vi "运维调试_其他.vi"() -> ()   [LabVIEW 2016, in "其他.lvlib"]
uses:
  <vilib>/Utility/miscctls.llb/LVPointTypeDef.ctl
  PLC/PLC.lvlib
  <vilib>/ptbypt/NI_PtbyPt.lvlib
panel:
  out "工作电流":dbl format="%#.2f A"
  out "工作电压":dbl format="%#.2f V"
  out "回风温度":dbl format="%#.2f ℃"
  out "空调通讯状态":u16(ring) items=["通讯异常", "通讯正常"]
  out "送风温度":dbl format="%#.2f ℃"
  out "集成报警信息":string
  out "R115":i16 caption="灯带关闭时间"
  out "R114":i16 caption="灯带开启时间"
  in  "视频监控":bool
  in  "照明":bool
  in  "前门灯带":bool
  in  "侧边灯带":bool
  # "空调运行状态"
  # "H"
  # "H"
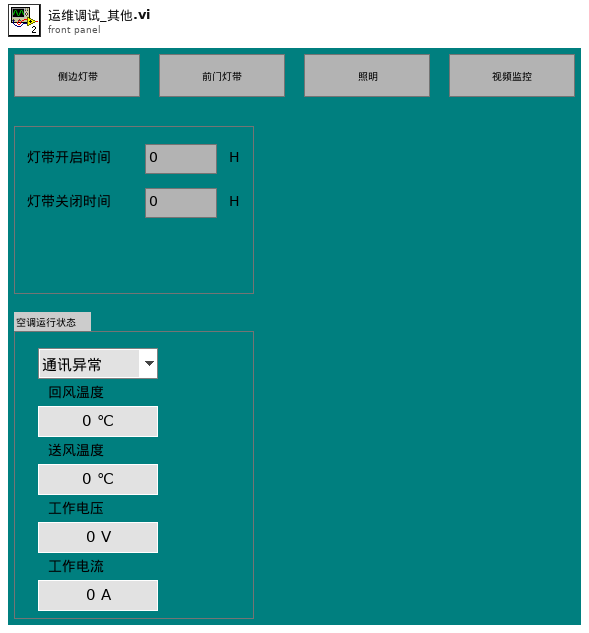
[diagram p1: front panel]
types:
  T1 = cluster{"通讯状态":u16, "回风温度":sgl, "送风温度":sgl, "电压":sgl, "电流":sgl}
  T2 = typedef "LVDateTimeRec.ctl" = cluster{"秒数的小数部分":dbl, "秒":i32, "分":i32, "时":i32, "日":i32, "月":i32, "年":i32, "天数（周）":i32, "天数（年）":i32, "DST":i32}
  T3 = cluster{"时间标识":timestamp, "监测值":sgl, "单位":string}
  T4 = cluster{"R100":i16, "R101":i16, "R102":i16, "R103":i16, "R104":i16, "R105":i16, "R106":i16, "R107":i16, "R108":i16, "R109":i16, "R110":i16, "R111":i16, "R112":i16, "R113":i16, "R114":i16, "R115":i16, "R116":i16, "R117":i16, "R118":i16, "R119":i16}
  T5 = typedef "LVPointTypeDef.ctl" = cluster{"Horizontal":i16, "Vertical":i16}
  T6 = cluster{"命令":string, "data":cluster{"starting address":u16, "coil values":bool[]}}
  T7 = cluster{"命令":string, "数据":cluster{"starting address":u16, "holding register values":u16[]}}
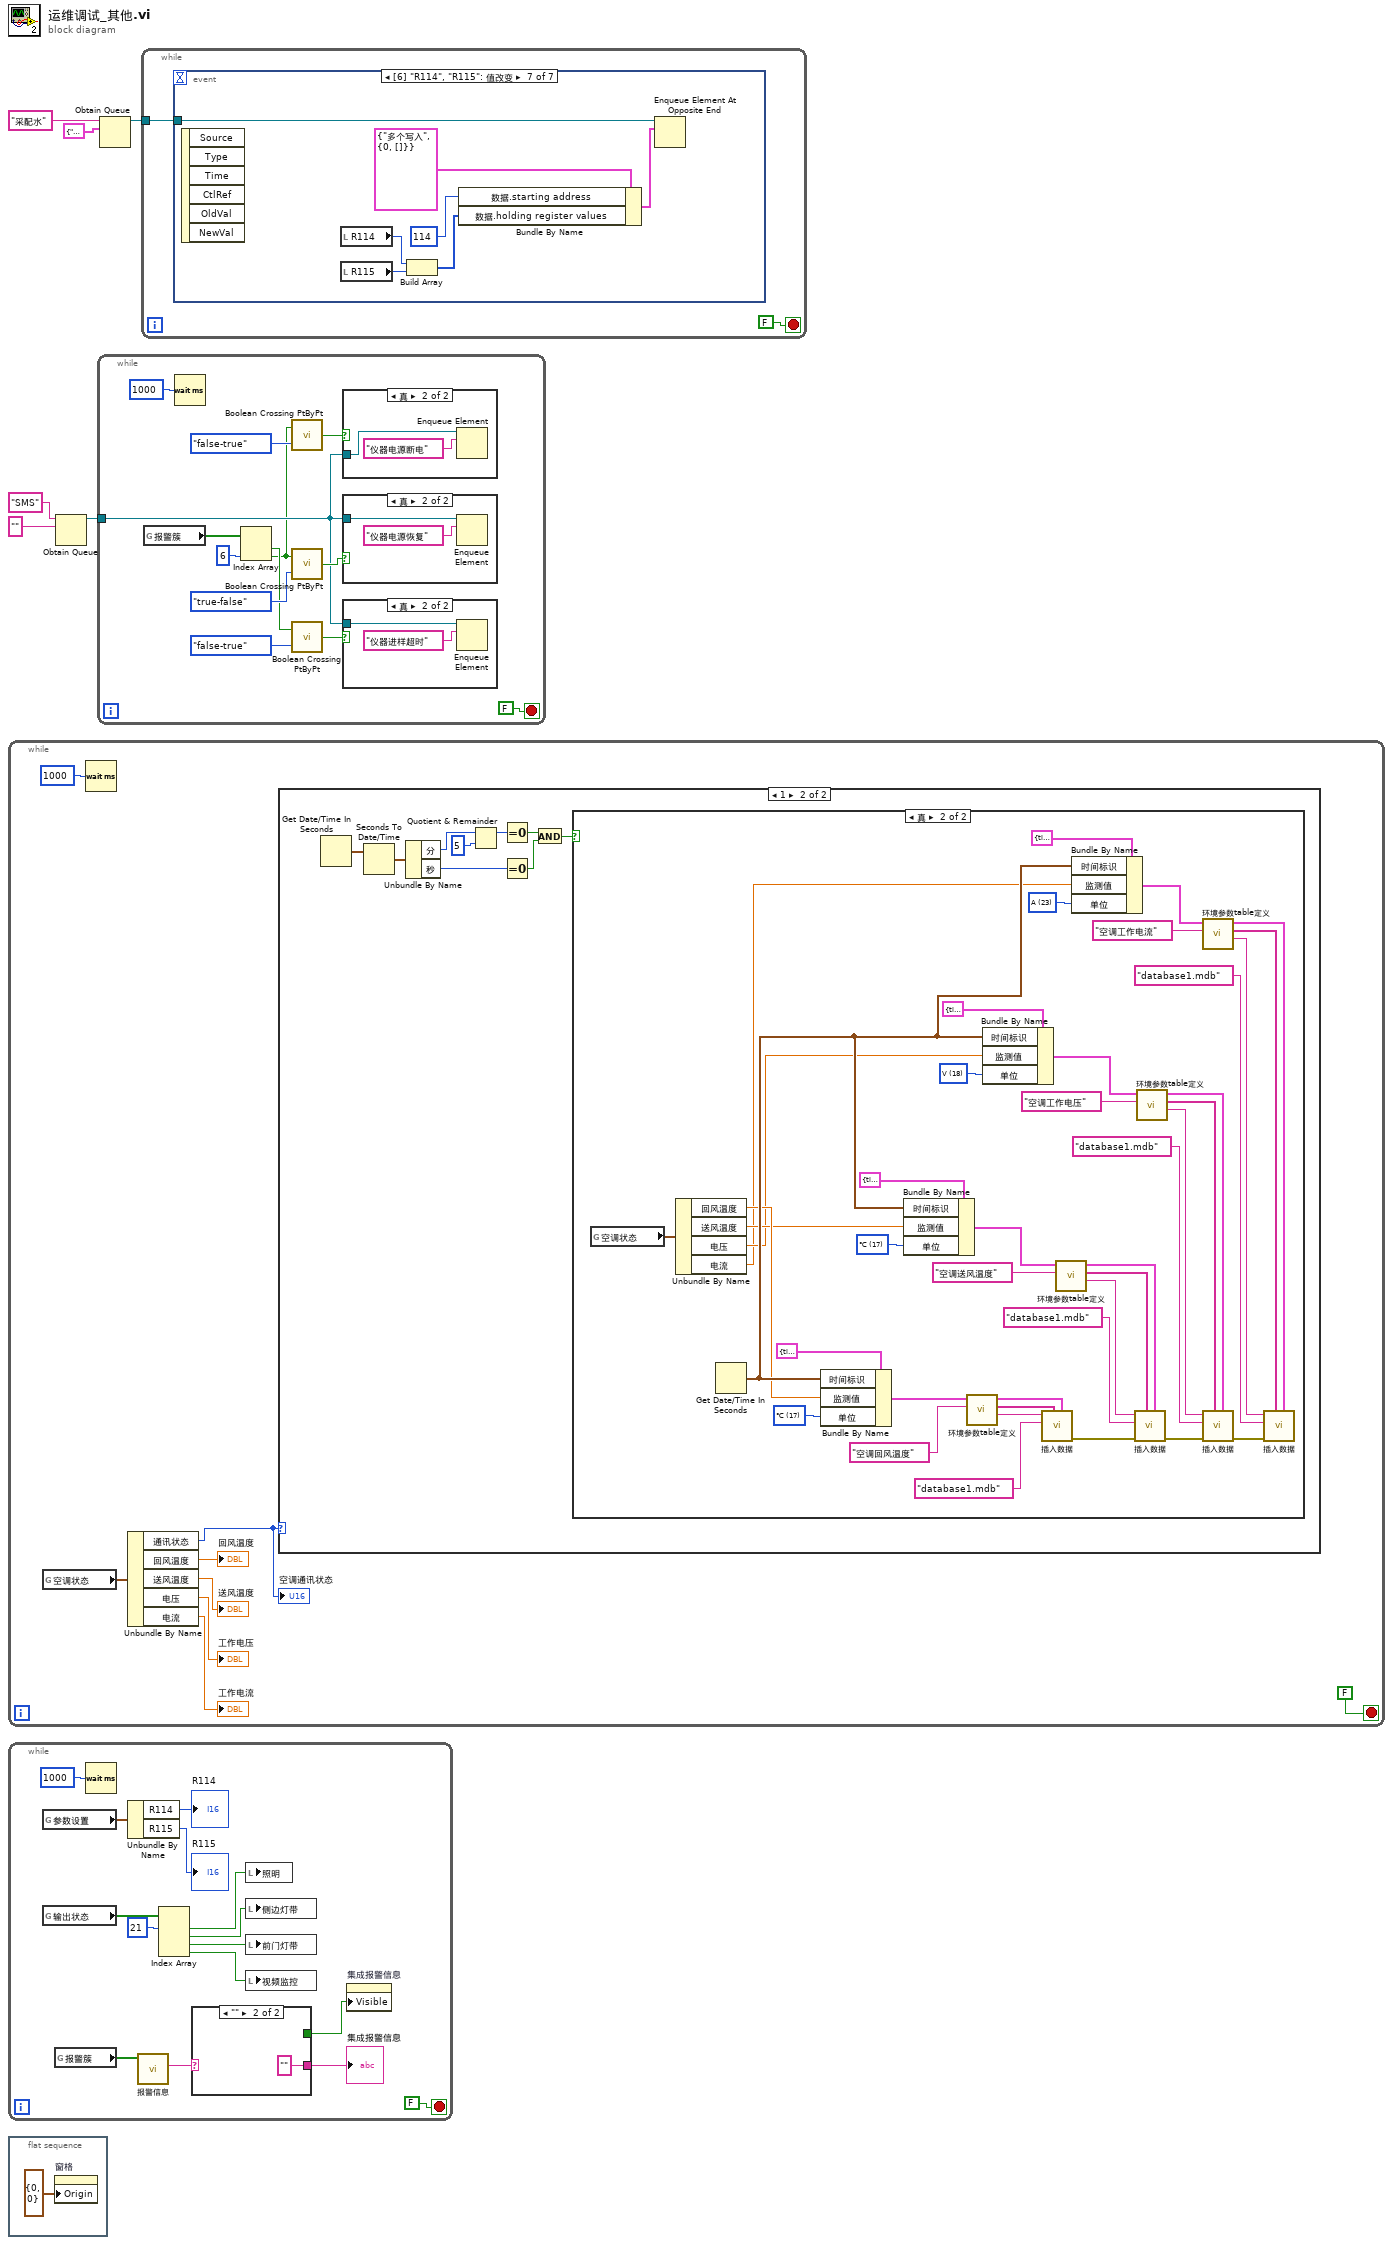
[diagram p0: block diagram]
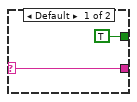
[diagram p7: hidden frame]
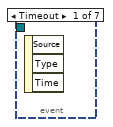
[diagram p8: hidden frame]
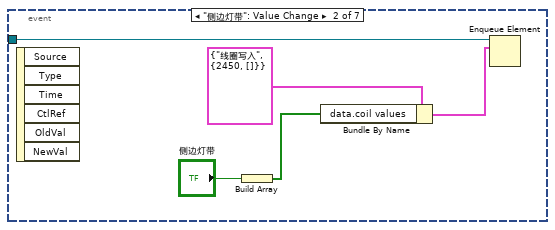
[diagram p9: hidden frame]
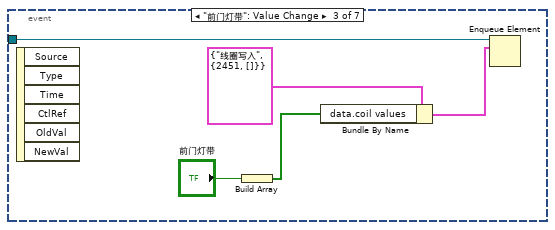
[diagram p10: hidden frame]
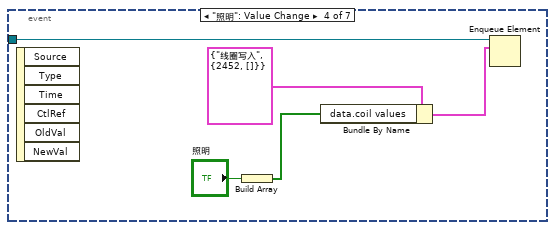
[diagram p11: hidden frame]
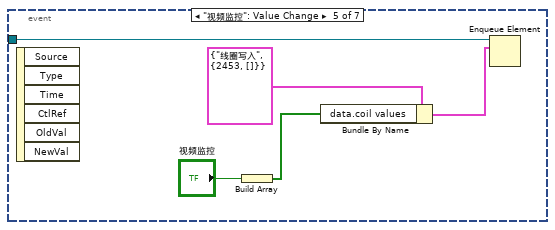
[diagram p12: hidden frame]
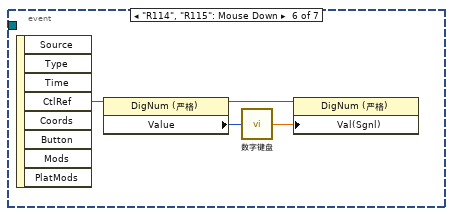
[diagram p13: hidden frame]
diagram:
  n1 = while {
    stop <- FALSE stop-if-true
    n2 = global read "采配水全局变量.vi" "空调状态"() -> (w14:T1)
    n3 = Wait (ms)(milliseconds to wait=u32 1000 ("等待时间（毫秒）")) -> ()  [unwired: 1 out]
    n4 = Unbundle By Name(w14) -> ("通讯状态"=w8:u16, "回风温度"=→"回风温度":sgl, "送风温度"=→"送风温度":sgl, "电压"=→"工作电压":sgl, "电流"=→"工作电流":sgl)
    "空调通讯状态" <- w8
    n5 = case shown="1" w8 {
      frame 0, Default {
      }
      frame 1 {
        n6 = Get Date/Time In Seconds() -> (seconds since 1Jan1904=w23:timestamp)
        n7 = Seconds To Date/Time(time stamp (now)=w23) -> (date time rec=w22:T2)  [unwired: 1 in]
        n8 = Unbundle By Name(w22) -> ("分"=w21:i32, "秒"=w19:i32)
        n9 = Quotient & Remainder(x=w21, y=5) -> (x-y*floor(x/y)=w18:i32)  [unwired: 1 out]
        n10 = Equal To 0?(x=w18) -> (x = 0?=w17:bool)
        n11 = Equal To 0?(x=w19) -> (x = 0?=w16:bool)
        n12 = And(x=w17, y=w16) -> (x .and. y?=w15:bool)
        n13 = case shown="真" w15 {
          frame False {
          }
          frame True {
            w29 = u16 23 items=["ug/L", "mg/L", "ppm", "mg/m3", "cm", "ppb", "ug/m3", "%", "nmol/mol", "umol/mol", "MPN/L", "MPN/100ml", "ng/m3", "NTU", "无量纲", "ms/cm", "us/cm", "℃", "V", "m3/s", "m3", "m", "m/s", "A"] ("单位")
            w45 = u16 18 items=["ug/L", "mg/L", "ppm", "mg/m3", "cm", "ppb", "ug/m3", "%", "nmol/mol", "umol/mol", "MPN/L", "MPN/100ml", "ng/m3", "NTU", "无量纲", "ms/cm", "us/cm", "℃", "V"] ("单位")
            w53 = u16 17 items=["ug/L", "mg/L", "ppm", "mg/m3", "cm", "ppb", "ug/m3", "%", "nmol/mol", "umol/mol", "MPN/L", "MPN/100ml", "ng/m3", "NTU", "无量纲", "ms/cm", "us/cm", "℃", "V"] ("单位")
            w55 = u16 17 items=["ug/L", "mg/L", "ppm", "mg/m3", "cm", "ppb", "ug/m3", "%", "nmol/mol", "umol/mol", "MPN/L", "MPN/100ml", "ng/m3", "NTU", "无量纲", "ms/cm", "us/cm", "℃", "V"] ("单位")
            n14 = global read "采配水全局变量.vi" "空调状态"() -> (w28:T1)
            n15 = Unbundle By Name(w28) -> ("回风温度"=w27:sgl, "送风温度"=w26:sgl, "电压"=w25:sgl, "电流"=w24:sgl)
            n16 = Get Date/Time In Seconds() -> (seconds since 1Jan1904=w30:timestamp)
            n17 = Bundle By Name(cluster=cluster{"时间标识":timestamp, "监测值":sgl, "单位":u16} {"时间标识"=timestamp(0 s since 1904-01-01), "监测值"=0.0, "单位"=0} ("data"), "时间标识"=w30, "监测值"=w27, "单位"=w55) -> (w56:cluster{"时间标识":timestamp, "监测值":sgl, "单位":u16})
            n18 = Bundle By Name(cluster=cluster{"时间标识":timestamp, "监测值":sgl, "单位":u16} {"时间标识"=timestamp(0 s since 1904-01-01), "监测值"=0.0, "单位"=0} ("data"), "时间标识"=w30, "监测值"=w26, "单位"=w53) -> (w52:cluster{"时间标识":timestamp, "监测值":sgl, "单位":u16})
            n19 = call "环境参数table定义.vi"("table 输入"="空调回风温度", "data"=w56) -> ("table 输出"=w64:string, "columns"=w63:string[], "data输出"=w62:T3)  [unwired: 7 in]
            n20 = Bundle By Name(cluster=cluster{"时间标识":timestamp, "监测值":sgl, "单位":u16} {"时间标识"=timestamp(0 s since 1904-01-01), "监测值"=0.0, "单位"=0} ("data"), "时间标识"=w30, "监测值"=w25, "单位"=w45) -> (w44:cluster{"时间标识":timestamp, "监测值":sgl, "单位":u16})
            n21 = call "插入数据.vi"("data"=w62, "columns"=w63, "database"="database1.mdb" ("table 输入"), "table"=w64) -> ("error out"=w58:errorcluster)  [unwired: 7 in]
            n22 = call "环境参数table定义.vi"("table 输入"="空调送风温度", "data"=w52) -> ("table 输出"=w59:string, "columns"=w60:string[], "data输出"=w61:T3)  [unwired: 7 in]
            n23 = Bundle By Name(cluster=cluster{"时间标识":timestamp, "监测值":sgl, "单位":u16} {"时间标识"=timestamp(0 s since 1904-01-01), "监测值"=0.0, "单位"=0} ("data"), "时间标识"=w30, "监测值"=w24, "单位"=w29) -> (w35:cluster{"时间标识":timestamp, "监测值":sgl, "单位":u16})
            n24 = call "插入数据.vi"("data"=w61, "columns"=w60, "error in (no error)"=w58, "database"="database1.mdb" ("table 输入"), "table"=w59) -> ("error out"=w32:errorcluster)  [unwired: 6 in]
            n25 = call "环境参数table定义.vi"("table 输入"="空调工作电压", "data"=w44) -> ("table 输出"=w40:string, "columns"=w41:string[], "data输出"=w42:T3)  [unwired: 7 in]
            n26 = call "环境参数table定义.vi"("table 输入"="空调工作电流", "data"=w35) -> ("table 输出"=w39:string, "columns"=w38:string[], "data输出"=w37:T3)  [unwired: 7 in]
            n27 = call "插入数据.vi"("data"=w42, "columns"=w41, "error in (no error)"=w32, "database"="database1.mdb" ("table 输入"), "table"=w40) -> ("error out"=w31:errorcluster)  [unwired: 6 in]
            n28 = call "插入数据.vi"("data"=w37, "columns"=w38, "error in (no error)"=w31, "database"="database1.mdb" ("table 输入"), "table"=w39) -> ()  [unwired: 6 in, 1 out]
          }
        }
      }
    }
  }
  n29 = while {
    stop <- FALSE stop-if-true
    n30 = global read "采配水全局变量.vi" "参数设置"() -> (w77:T4)
    n31 = global read "采配水全局变量.vi" "输出状态"() -> (w70:bool[])
    n32 = global read "采配水全局变量.vi" "报警簇"() -> (w71:bool[])
    n33 = Wait (ms)(milliseconds to wait=u32 1000 ("等待时间（毫秒）")) -> ()  [unwired: 1 out]
    n34 = Unbundle By Name(w77) -> ("R114"=→"R114":i16, "R115"=→"R115":i16)
    n35 = call "报警信息.vi"("报警簇"=w71) -> ("系统报警信息"=w74:string)  [unwired: 9 in, 1 out]
    n36 = Index Array(array=w70, index #1=21 ("索引")) -> (element #1=w68:bool, element #2=w67:bool, element #3=w69:bool, element #4=w66:bool)  [unwired: 3 in]
    n37 = case shown="\"\"" w74 {
      selector: w74 -> [w81 _]
      tunnel: [w81 "" ("字符串")] -> w72
      tunnel: [TRUE ("可见") _] -> w73
      frame Default {
      }
      frame "" {
      }
    }
    "集成报警信息" <- w72
    n38 = local write "照明"(w68) -> ()
    n39 = local write "侧边灯带"(w67) -> ()
    n40 = local write "前门灯带"(w69) -> ()
    n41 = local write "视频监控"(w66) -> ()
    n42 = property on="集成报警信息" class="Str"("Visible"=w73) -> ()  [unwired: 2 in, 2 out]
  }
  n43 = flat-sequence {
    frame #0 {
      n44 = property on="窗格" class="Pane"("Origin"=T5 {"Horizontal"=0, "Vertical"=0} ("原点")) -> ()  [unwired: 2 in, 2 out]
    }
  }
  n45 = Obtain Queue(name (unnamed)="SMS" ("名称（未命名）"), element data type="" ("名称（未命名）")) -> (queue out=w1:refnum<queue>)  [unwired: 3 in, 2 out]
  n46 = while {
    tunnel: w1 -> [w90]
    stop <- FALSE stop-if-true
    n47 = global read "采配水全局变量.vi" "报警簇"() -> (w87:bool[])
    n48 = Wait (ms)(milliseconds to wait=u32 1000 ("等待时间（毫秒）")) -> ()  [unwired: 1 out]
    n49 = Index Array(array=w87, index #2=6 ("索引")) -> (element #1=w86:bool, element #2=w84:bool)  [unwired: 1 in]
    n50 = call <vilib>:"Boolean Crossing PtByPt.vi"("direction"=enum16{"either", "false-true", "true-false"}."false-true", "input"=w84) -> ("crossing"=w93:bool)  [unwired: 1 in]
    n51 = call <vilib>:"Boolean Crossing PtByPt.vi"("direction"=enum16{"either", "false-true", "true-false"}."true-false", "input"=w84) -> ("crossing"=w91:bool)  [unwired: 1 in]
    n52 = call <vilib>:"Boolean Crossing PtByPt.vi"("direction"=enum16{"either", "false-true", "true-false"}."false-true", "input"=w86) -> ("crossing"=w88:bool)  [unwired: 1 in]
    n53 = case shown="真" w93 {
      tunnel: w90 -> [_ w102]
      frame False {
      }
      frame True {
        n54 = Enqueue Element(queue=w102, element="仪器电源断电" ("元素")) -> ()  [unwired: 2 in, 3 out]
      }
    }
    n55 = case shown="真" w91 {
      tunnel: w90 -> [_ w100]
      frame False {
      }
      frame True {
        n56 = Enqueue Element(queue=w100, element="仪器电源恢复" ("元素")) -> ()  [unwired: 2 in, 3 out]
      }
    }
    n57 = case shown="真" w88 {
      tunnel: w90 -> [_ w98]
      frame False {
      }
      frame True {
        n58 = Enqueue Element(queue=w98, element="仪器进样超时" ("元素")) -> ()  [unwired: 2 in, 3 out]
      }
    }
  }
  n59 = Obtain Queue(name (unnamed)="采配水" ("名称（未命名）"), element data type=cluster{"命令":string, "数据":variant} {"命令"="", "数据"=variant}) -> (queue out=w4:refnum<queue>)  [unwired: 3 in, 2 out]
  n60 = while {
    tunnel: w4 -> [w103]
    stop <- FALSE stop-if-true
    n61 = event shown="[6] \"R114\", \"R115\": 值改变" {
      selector: _ -> [_ _ _ _ _ _ _]
      dyn-events: _ -> [_ _ _ _ _ _ _]
      timeout: _ -> [_ _ _ _ _ _ _]
      tunnel: w103 -> [_ w106 w112 w117 w122 _ w129]
      event Timeout {
        n62 = event-data() -> ()  [unwired: 1 in, 3 out]
      }
      event "侧边灯带": Value Change {
        n63 = event-data() -> ()  [unwired: 1 in, 6 out]
        n64 = Build Array("侧边灯带") -> (w105:bool[])
        n65 = Bundle By Name(cluster=T6 {"命令"="线圈写入", "data"={"starting address"=2450, "coil values"=[]}} ("元素"), "data.coil values"=w105) -> (w107:T6)
        n66 = Enqueue Element(queue=w106, element=w107) -> ()  [unwired: 2 in, 3 out]
      }
      event "前门灯带": Value Change {
        n67 = event-data() -> ()  [unwired: 1 in, 6 out]
        n68 = Build Array("前门灯带") -> (w111:bool[])
        n69 = Bundle By Name(cluster=T6 {"命令"="线圈写入", "data"={"starting address"=2451, "coil values"=[]}} ("元素"), "data.coil values"=w111) -> (w113:T6)
        n70 = Enqueue Element(queue=w112, element=w113) -> ()  [unwired: 2 in, 3 out]
      }
      event "照明": Value Change {
        n71 = event-data() -> ()  [unwired: 1 in, 6 out]
        n72 = Build Array("照明") -> (w116:bool[])
        n73 = Bundle By Name(cluster=T6 {"命令"="线圈写入", "data"={"starting address"=2452, "coil values"=[]}} ("元素"), "data.coil values"=w116) -> (w118:T6)
        n74 = Enqueue Element(queue=w117, element=w118) -> ()  [unwired: 2 in, 3 out]
      }
      event "视频监控": Value Change {
        n75 = event-data() -> ()  [unwired: 1 in, 6 out]
        n76 = Build Array("视频监控") -> (w121:bool[])
        n77 = Bundle By Name(cluster=T6 {"命令"="线圈写入", "data"={"starting address"=2453, "coil values"=[]}} ("元素"), "data.coil values"=w121) -> (w123:T6)
        n78 = Enqueue Element(queue=w122, element=w123) -> ()  [unwired: 2 in, 3 out]
      }
      event "R114", "R115": Mouse Down {
        n79 = event-data() -> ("CtlRef"=w128:refnum<vi>)  [unwired: 1 in, 7 out]
        n80 = property class="DigNum (严格)"(reference=w128) -> (reference out=w127:refnum<vi>, "Value"=w126:i16)  [unwired: 1 in, 1 out]
        n81 = call "数字键盘.vi"("OldNumber"=w126) -> ("NewNumber"=w125:sgl)
        n82 = property class="DigNum (严格)"(reference=w127, "Val(Sgnl)"=w125) -> ()  [unwired: 1 in, 2 out]
      }
      event "R114", "R115": Value Change {
        n83 = event-data() -> ()  [unwired: 1 in, 6 out]
        n84 = local read "R114"() -> (w134:i16)
        n85 = local read "R115"() -> (w135:i16)
        n86 = Build Array(w134, w135) -> (w130:i16[])
        n87 = Bundle By Name(cluster=T7 {"命令"="多个写入", "数据"={"starting address"=0, "holding register values"=[]}} ("元素"), "数据.starting address"=u16 114, "数据.holding register values"=w130) -> (w131:T7)
        n88 = Enqueue Element At Opposite End(queue=w129, element=w131) -> ()  [unwired: 2 in, 3 out]
      }
    }
  }
